vi "strainGaugeTester.vi"() -> ()   [LabVIEW 2012]
uses:
  <vilib>/DAQmx/read.llb/DAQmx Read (Analog 1D DBL 1Chan NSamp).vi
  <vilib>/DAQmx/create/channels.llb/DAQmx Create Channel (AI-Voltage-Basic).vi
  <vilib>/DAQmx/configure/timing.llb/DAQmx Timing (Sample Clock).vi
  <vilib>/DAQmx/miscellaneous.llb/DAQmx Fill In Error Info.vi
panel:
  out "mass":dbl format="%#.3g"
  out "Force(N)":dbl format="%#.3g"
  in  "Bias":bool
  out "Voltages":dbl format="%#.3g"
  in  "stop":bool
  in  "Timing parameters":T1={"Sample Rate"=1000.0, "Samples to Read"=100}
  in  "physical channels":tag
  out "Measurement":dbl[](graph) caption="F/T Data"
  in  "bias":dbl format="%#.3g"
  out "error out":errorcluster
  in  "error in":errorcluster
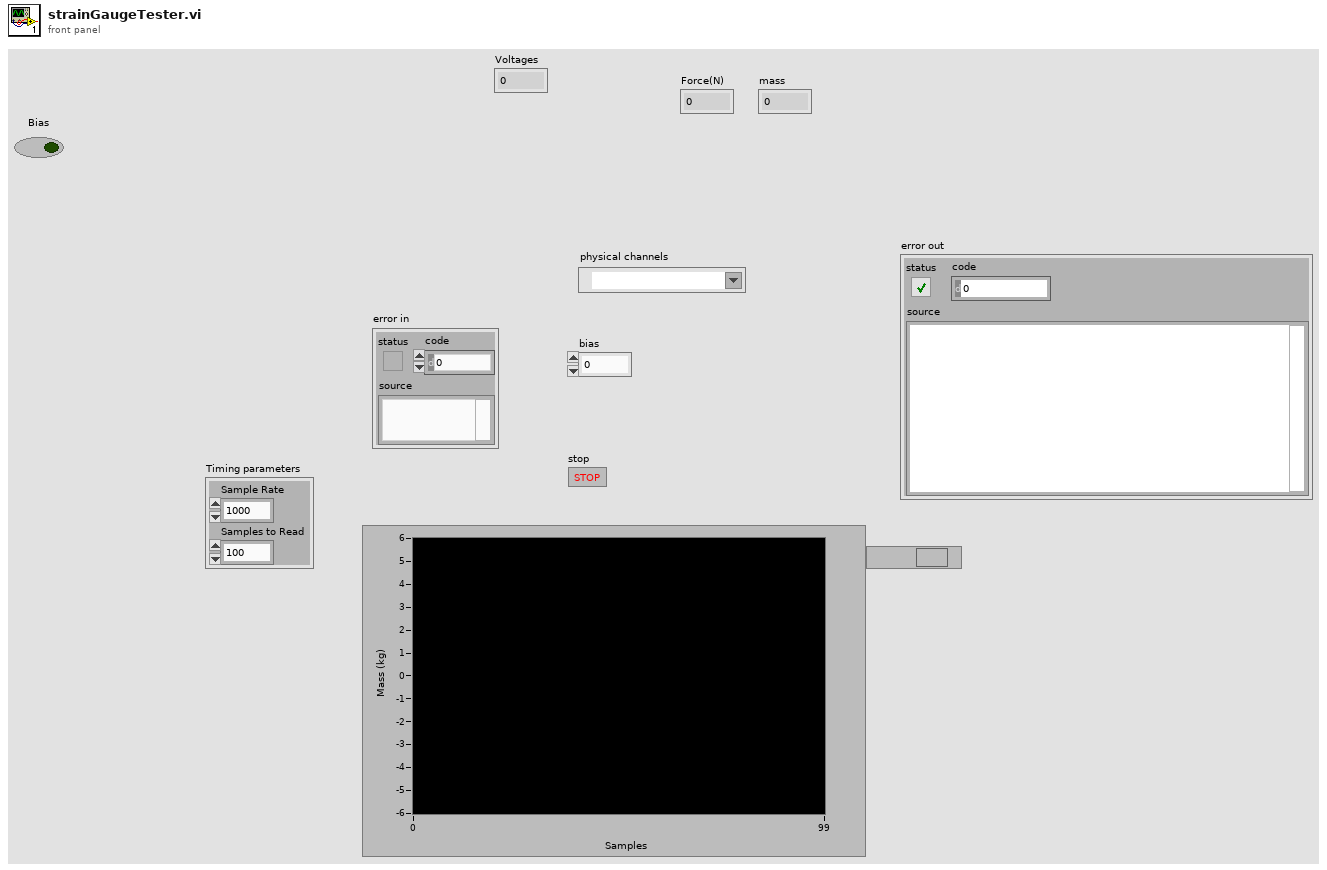
[diagram p1: front panel]
types:
  T1 = cluster{"Sample Rate":dbl, "Samples to Read":i32}
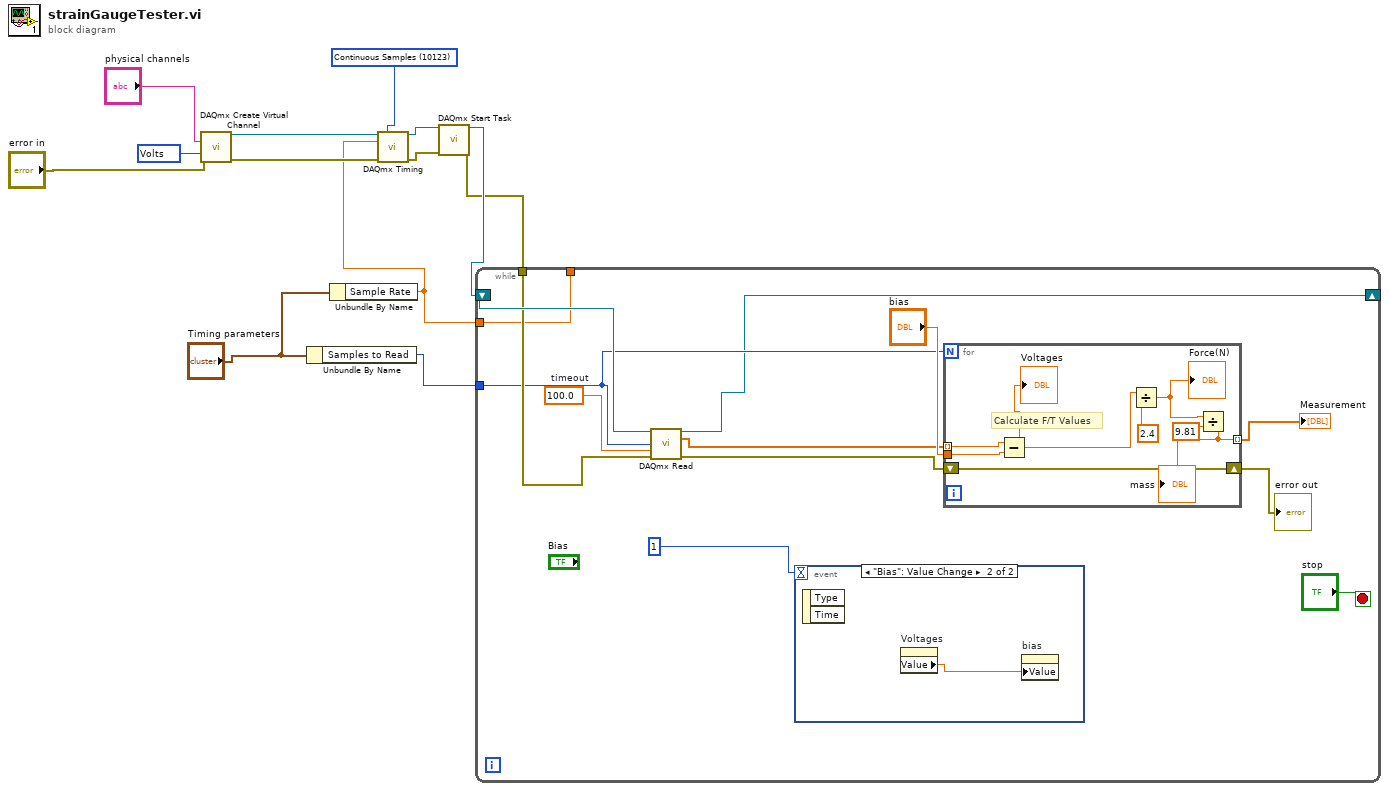
[diagram p0: block diagram]
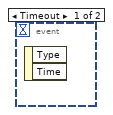
[diagram p2: hidden frame]
diagram:
  w1 = 10123 items=["Finite Samples"=10178, "Continuous Samples"=10123] ("sample mode")
  w10 = 10348 items=["Volts"=10348, "From Custom Scale"=10065] ("units")
  n1 = call-poly <vilib>:"DAQmx Create Virtual Channel.vi"("physical channels"="physical channels", "units"=w10, "error in"="error in") -> ("task out"=w13:refnum<k21>, "error out"=w12:errorcluster)  [unwired: 11 in]
  n2 = Unbundle By Name("Timing parameters") -> ("Samples to Read"=w3:i32)
  n3 = Unbundle By Name("Timing parameters") -> ("Sample Rate"=w2:dbl)
  n4 = call-poly <vilib>:"DAQmx Timing.vi"("task/channels in"=w13, "sample mode"=w1, "rate"=w2, "error in"=w12) -> ("task out"=w6:refnum<k21>, "error out"=w8:errorcluster)  [unwired: 10 in]
  n5 = call <vilib>:"DAQmx Start Task.vi"("task/channels in"=w6, "error in"=w8) -> ("task out"=w9:refnum<k21>, "error out"=w5:errorcluster)  [unwired: 12 in]
  n6 = while {
    tunnel: [w19] -> _
    tunnel: w5 -> [w24]
    tunnel: w3 -> [w20]
    tunnel: w2 -> [w19]
    shift-right: [w17] -> _
    shift-left: w9 -> [w25]
    stop <- "stop" stop-if-true
    w26 = 100.0  # timeout
    n7 = call-poly <vilib>:"DAQmx Read.vi"("task/channels in"=w25, "number of samples per channel"=w20, "timeout"=w26, "error in"=w24) -> ("task out"=w17:refnum<k21>, "data"=w15:dbl[], "error out"=w22:errorcluster)  [unwired: 9 in]
    n8 = event shown="[1] \"Bias\": Value Change" {
      selector: _ -> [_ _]
      dyn-events: _ -> [_ _]
      timeout: 1 -> [_ _]
      event Timeout {
        n9 = event-data() -> ()  [unwired: 1 in, 2 out]
      }
      event "Bias": Value Change {
        n10 = event-data() -> ()  [unwired: 1 in, 2 out]
        n11 = property on="Voltages" class="DigNum (strict)"() -> ("Value"=w27:dbl)  [unwired: 2 in, 2 out]
        n12 = property on="bias" class="DigNum (strict)"("Value"=w27) -> ()  [unwired: 2 in, 2 out]
      }
    }
    n13 = for {
      N: w20 -> [_]
      shift-right: [w35] -> w21
      shift-left: w22 -> [w35]
      tunnel: "bias" -> [w34]
      tunnel: w15 -> [w33] mode=indexing
      tunnel: [w29] -> w16 mode=indexing
      # "Calculate F/T Values"
      n14 = Subtract(x=w33, y=w34) -> (x-y=w32:dbl)
      "Voltages" <- w32
      n15 = Divide(x=w32, y=2.4) -> (x/y=w30:dbl)
      "Force(N)" <- w30
      n16 = Divide(x=w30, y=9.81) -> (x/y=w29:dbl)
      "mass" <- w29
    }
    "error out" <- w21
    "Measurement" <- w16
  }
